vi "ex15-2.vi"() -> ()   [LabVIEW 2013]
uses:
  <vilib>/University of Leeds/Kinesthesia Toolkit for Microsoft Kinect/_Polymorphic Configure/Event-Skeleton.vi
  <vilib>/University of Leeds/Kinesthesia Toolkit for Microsoft Kinect/_Polymorphic Close/Close-Skeleton.vi
  <vilib>/University of Leeds/Kinesthesia Toolkit for Microsoft Kinect/_Polymorphic Read/Read-Skeleton.vi
panel:
  in  "stop":bool
  out "3D Picture":refnum<vi>(3d-picture)
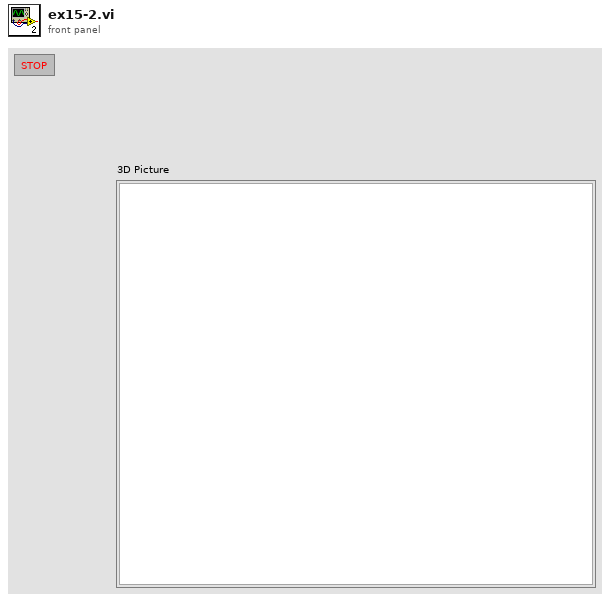
[diagram p1: front panel]
types:
  T1 = cluster{cluster{"reference out":refnum<k24>, "KinectSensors":refnum<k24>}, "get_Item":refnum<k24>}
  T2 = cluster{"reference out":refnum<k24>, "KinectSensors":refnum<k24>, "SkeletonStream":refnum<k24>, refnum<k24>[], "get_Item":refnum<k24>}
  T3 = cluster{"Scene":refnum<vi>, "Joints":refnum<vi>[], "Bones":refnum<vi>[]}
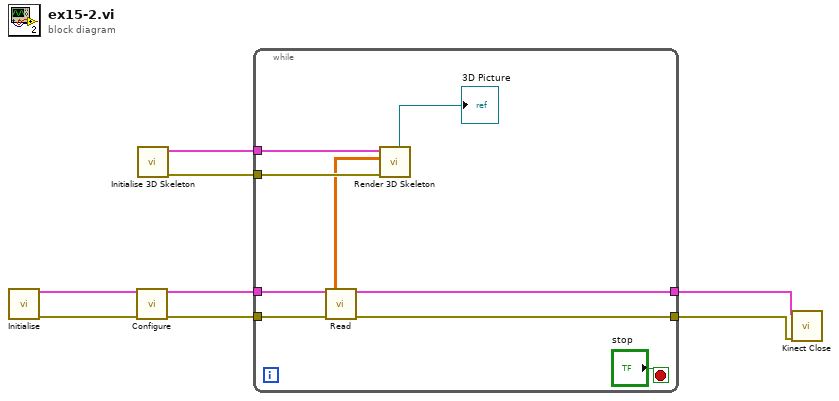
[diagram p0: block diagram]
diagram:
  n1 = call <vilib>:"Initialise.vi"() -> ("Kinect References out"=w8:T1, "error out"=w7:errorcluster)  [unwired: 14 in]
  n2 = call-poly <vilib>:"Configure.vi"("Kinect References in"=w8, "error in"=w7) -> ("Kinect References out"=w6:T2, "error out"=w5:errorcluster)  [unwired: 12 in]
  n3 = call <vilib>:"Initialise 3D Skeleton.vi"() -> ("error out"=w3:errorcluster, "Scene & Skeleton Refs"=w4:T3)  [unwired: 10 in]
  n4 = while {
    tunnel: w6 -> [w17]
    tunnel: w5 -> [w16]
    tunnel: w4 -> [w15]
    tunnel: w3 -> [w14]
    tunnel: [w11] -> w2
    tunnel: [w10] -> w1
    stop <- "stop" stop-if-true
    n5 = call-poly <vilib>:"Read.vi"("Kinect References in"=w17, "error in (no error)"=w16) -> ("Primary Skeleton Array"=w9:dbl[][], "Kinect References out"=w11:T2, "error out"=w10:errorcluster)  [unwired: 10 in, 1 out]
    n6 = call <vilib>:"Render 3D Skeleton.vi"("error in (no error)"=w14, "Array of Joint Positions"=w9, "Scene & Skeleton Refs In"=w15) -> ("Scene Out"=→"3D Picture":refnum<vi>)  [unwired: 5 in, 3 out]
  }
  n7 = call-poly <vilib>:"Kinect Close.vi"("Kinect References in"=w2, "error in"=w1) -> ()  [unwired: 13 in, 1 out]
